vi "CLC_L2_8x8_InPhaseCal_L1_2x2_Auto16AiP.vi"() -> ()   [LabVIEW 2023, in "Clover_Cell.lvlib"]
uses:
  lib/CTL/AiP_index.ctl
  Clover_Cell.lvlib
  lib/Anritsu Signal Analyzer Series/Anritsu Signal Analyzer Series.lvlib
panel:
  out "Numeric":i32
  out "AiP_Change":i32
  out "FileNAME_Dual 2":string
  out "maxPower":dbl
  out "B_Ch_Index":i32[](array[numeric])
  out "A_Ch_Index":i32[](array[numeric])
  out "A-Phase":i32[](array[numeric])
  out "B-Phase":i32[](array[numeric])
  out "Duration(sec)":dbl
  out "Start":u32
  in  "AiP_Base":T1=1 items=["AiP_1"=1, "AiP_2"=2, "AiP_3"=3, "AiP_4"=4, "AiP_5"=5, "AiP_6"=6, "AiP_7"=7, "AiP_8"=8, "AiP_9"=9, "AiP_10"=10, "AiP_11"=11, "AiP_12"=12, "AiP_13"=13, "AiP_14"=14, "AiP_15"=15, "AiP_16"=16]
  in  "WaitingTime":u32=500
  in  "Polarity":u16(ring) items=["H", "V"]
  in  "AvgTimes":i32=5
  in  "TRXmode":u16(ring)=1 items=["Rx"=2, "Tx"=1]
  in  "FileName_Note":string
  out "AiP_Base_Ch":i32
  out "AiP_Change_OFFSetPhase":i32
  out "AiP_Change_Ch":i32
  out "max index\n(OFFSet Step)":i32
  out "trmode":u16
  in  "VISA resource name":refnum<visa-resource-name>="TCPIP0::192.168.100.230::inst0::INSTR"
  out "FileNAME_Dual":string
  out "OK?":bool
  out "output cluster":T2={"address"="192.168.100.111", "remote port or service name"=5025, "timeout ms (60000)"=10000}
  out "SA1":dbl[](graph)
  out "error out":errorcluster
  # "CLC_Gen3_L2_8x8_InPhase_Calibration_by_L1_2x2 Auto"
  # "Setting"
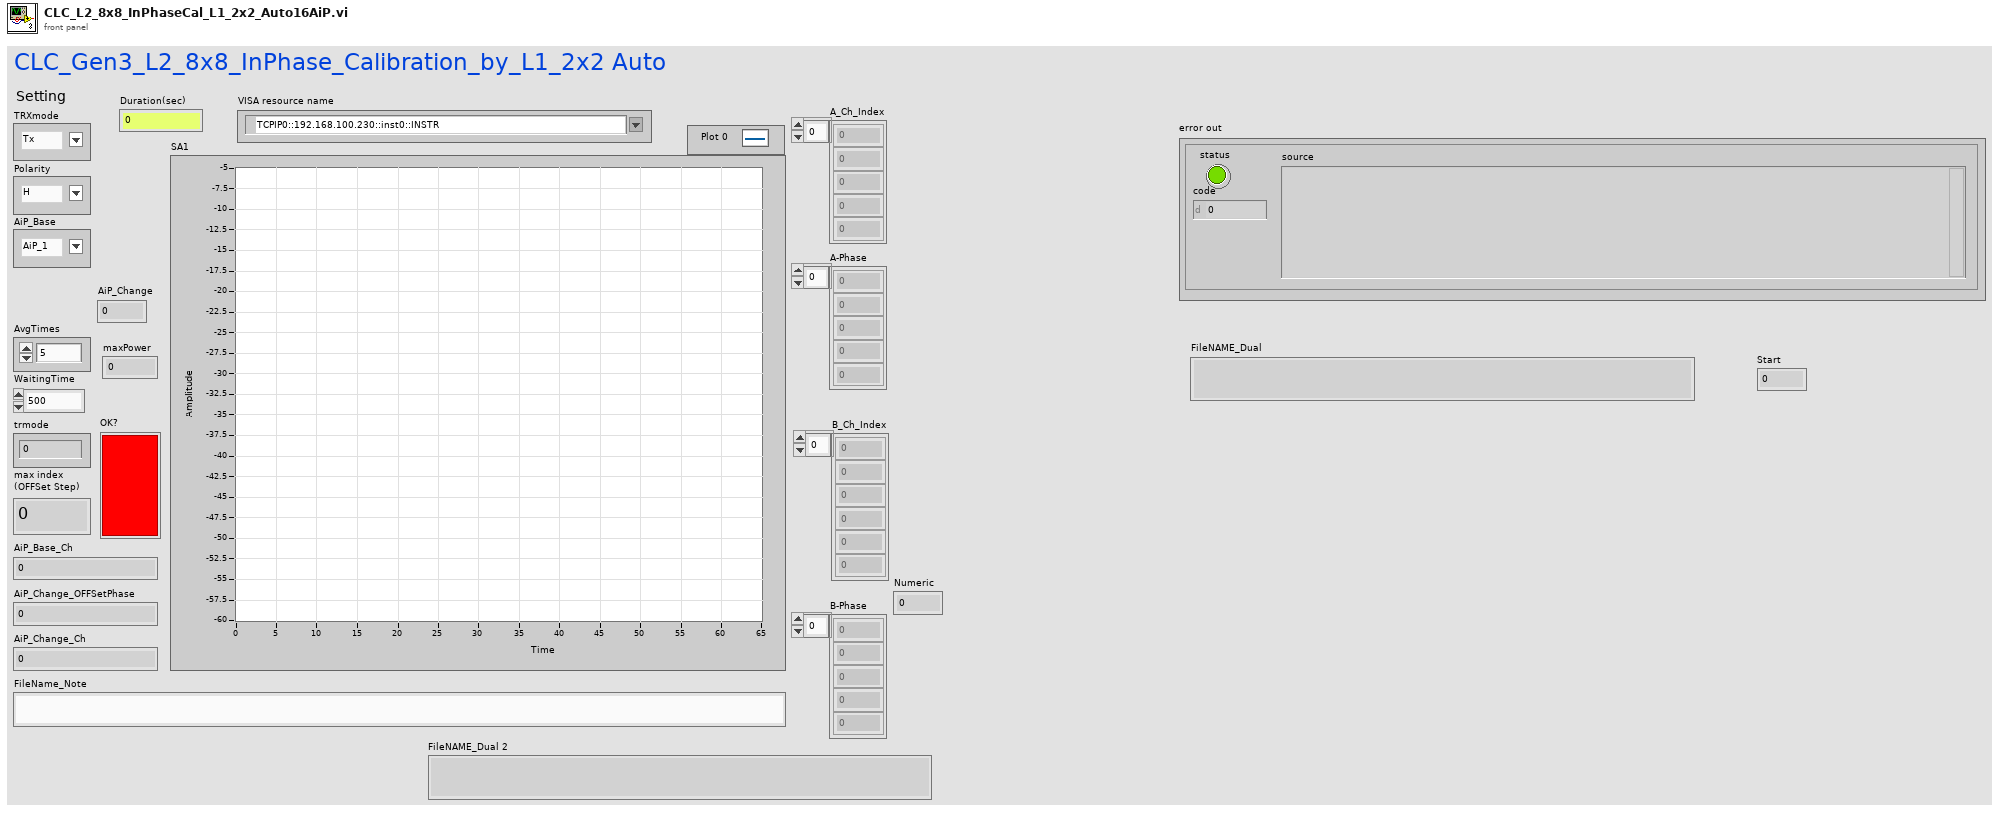
[diagram p1: front panel]
types:
  T1 = typedef "AiP_index.ctl" = u16
  T2 = cluster{"address":string, "remote port or service name":u16, "timeout ms (60000)":i32}
  T3 = cluster{"Mode":u16, "Polarity":u16, "CH_ON/OFF":u16, "Channel":i32, "Gain":i32, "Phase":i32}
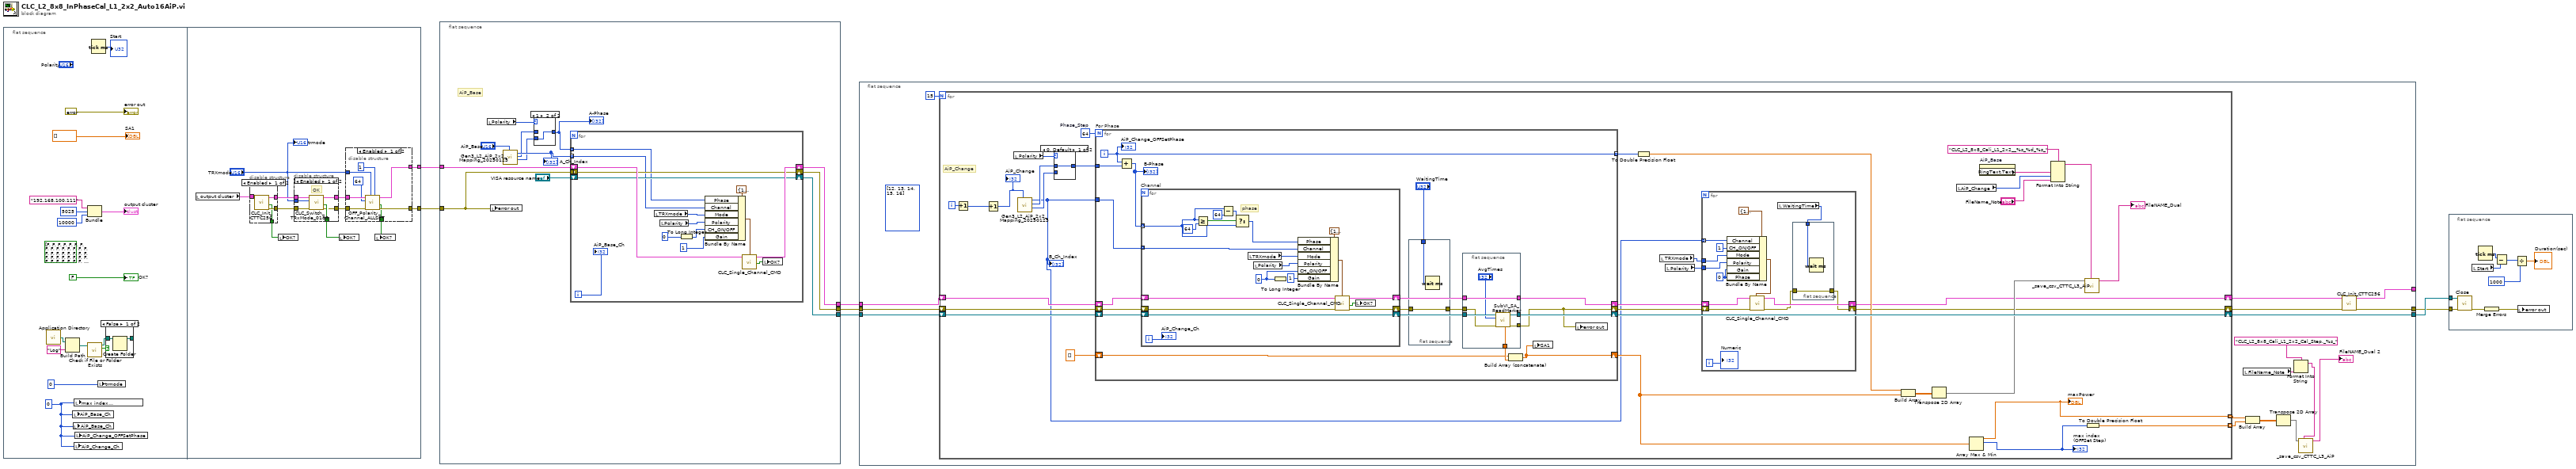
[diagram p0: block diagram]
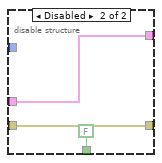
[diagram p5: hidden frame]
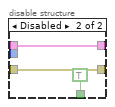
[diagram p6: hidden frame]
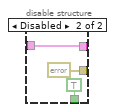
[diagram p7: hidden frame]
diagram:
  n1 = flat-sequence {
    tunnel: [w26] -> w1
    tunnel: [w31] -> w2
    frame #0 {
      w9 = 0 ("max index\n(OFFSet Step)")
      (unwired) bool[][] [[FALSE, FALSE, FALSE, FALSE, FALSE, FALSE, FALSE, FALSE], [FALSE, FALSE, FALSE, FALSE, FALSE, FALSE, FALSE, FALSE], [FALSE, FALSE, FALSE, FALSE, FALSE, FALSE, FALSE, FALSE], [FALSE, FALSE, FALSE, FALSE, FALSE, FALSE, FALSE, FALSE], [FALSE, FALSE, FALSE, FALSE, FALSE, FALSE, FALSE, FALSE], [FALSE, FALSE, FALSE, FALSE, FALSE, FALSE, FALSE, FALSE], [FALSE, FALSE, FALSE, FALSE, FALSE, FALSE, FALSE, FALSE], [FALSE, FALSE, FALSE, FALSE, FALSE, FALSE, FALSE, FALSE]] ("Operating \nChannel(s)")
      n2 = call <vilib>:"Application Directory.vi"() -> ("Application Directory"=w14:path)
      n3 = Build Path(base path=w14, name or relative path="Log") -> (appended path=w11:path)
      n4 = local write "AiP_Base_Ch"(w9) -> ()
      n5 = local write "AiP_Base_Ch"(w9) -> ()
      n6 = local write "AiP_Change_Ch"(w9) -> ()
      n7 = local write "max index\n(OFFSet Step)"(w9) -> ()
      n8 = local write "AiP_Change_OFFSetPhase"(w9) -> ()
      n9 = Bundle("address"="192.168.100.111", "remote port or service name"=u16 5025, "timeout ms (60000)"=10000) -> (→"output cluster":T2)  [unwired: 1 in]
      n10 = call <vilib>:"Check if File or Folder Exists.vi"("path"=w11) -> ("file or folder exists?"=w13:bool, "dup path"=w12:path)  [unwired: 8 in, 1 out]
      n11 = Tick Count (ms)() -> (millisecond timer value=→"Start":u32)
      n12 = local write "trmode"(u16 0 ("trmode")) -> ()
      n13 = case shown="False" w13 {
        tunnel: w12 -> [w24 w25]
        tunnel: [w23 w25] -> _
        frame False {
          n14 = Create Folder(path (use dialog)=w24) -> (created path=w23:path)  [unwired: 2 in, 2 out]
        }
        frame True {
        }
      }
      "error out" <- errorcluster {"status"=FALSE, "code"=0, "source"=""} ("error out")
      "OK?" <- FALSE ("OK?")
      "SA1" <- dbl[] []
    }
    frame #1 {
      n15 = local read "output cluster"() -> (w36:T2)
      n16 = disable-structure shown="Enabled" {
        disable-tunnel: w36 -> [w60 w63]
        disable-tunnel: [w59 w63] -> w35
        disable-tunnel: [w58 errorcluster {"status"=FALSE, "code"=0, "source"=""} ("error in (no error)")] -> w33
        disable-tunnel: [w57 TRUE ("OK?")] -> w28
        frame Enabled {
          n17 = call "CLC_Init_CTTC256.vi"("TCPIPin"=w60) -> ("error out"=w58:errorcluster, "Status"=w57:bool, "TCPIPin 2"=w59:T2)  [unwired: 8 in]
        }
        frame Disabled {
        }
      }
      n18 = local write "OK?"(w28) -> ()
      n19 = disable-structure shown="Enabled" {
        disable-tunnel: w35 -> [w53 w55]
        disable-tunnel: [w52 TRUE ("OK?")] -> w34
        disable-tunnel: w33 -> [w51 w54]
        disable-tunnel: [w50 w54] -> w32
        disable-tunnel: [w49 w55] -> w30
        disable-tunnel: "TRXmode" -> [w48 _]
        frame Enabled {
          # "OK"
          n20 = call "CLC_Switch_TRxMode_0188.vi"("error in (no error)"=w51, "Text Ring"=w48, "TCPIPin"=w53) -> ("error out"=w50:errorcluster, "OK?"=w52:bool, "TCPIPin 2"=w49:T2)  [unwired: 6 in]
        }
        frame Disabled {
        }
      }
      n21 = local write "OK?"(w34) -> ()
      n22 = disable-structure shown="Enabled" {
        disable-tunnel: w32 -> [w44 w46]
        disable-tunnel: [w43 w46] -> w31
        disable-tunnel: w30 -> [w42 w45]
        disable-tunnel: [w41 FALSE ("OK?")] -> w29
        disable-tunnel: "TRXmode" -> [w39 _]
        disable-tunnel: [w37 w45] -> w26
        frame Enabled {
          n23 = call "OFF_Polarity_Channel_ALLSET.vi"("CH_ON:0/OFF:1"=u16 1, "Mode"=w39, "error in"=w44, "Channel"=64, "TCPIPin"=w42) -> ("error out"=w43:errorcluster, "OK?"=w41:bool, "TCPIPout"=w37:T2)  [unwired: 4 in]
        }
        frame Disabled {
        }
      }
      n24 = local write "OK?"(w29) -> ()
      "trmode" <- "TRXmode"
    }
  }
  n25 = flat-sequence {
    tunnel: [w75] -> w7
    tunnel: [w74] -> w6
    tunnel: [w73] -> w5
    tunnel: w2 -> [w72]
    tunnel: w1 -> [w70]
    frame #0 {
      # "AiP_Base"
      n26 = local read "Polarity"() -> (w69:u16)
      n27 = local write "error out"(w72) -> ()
      n28 = call "Gen3_L2_AiP_2x2_Mapping_20250125.vi"("AiP"="AiP_Base") -> ("Pol_V"=w66:i32[], "Pol_H"=w67:i32[], "Ch_Index"=w68:i32[])  [unwired: 8 in]
      "A_Ch_Index" <- w68
      n29 = case shown="1" w69 {
        tunnel: w67 -> [w76 _]
        tunnel: [w76 w77] -> w64
        tunnel: w66 -> [_ w77]
        frame 0, Default {
        }
        frame 1 {
        }
      }
      "A-Phase" <- w64
      n30 = for {
        shift-right: [w89] -> w73
        shift-left: w70 -> [w88]
        tunnel: w72 -> [w83]
        shift-right: [w83] -> w74
        shift-left: _ -> [_]
        shift-right: [w82] -> w75
        shift-left: "VISA resource name" -> [w82]
        tunnel: w68 -> [w81] mode=indexing
        tunnel: w64 -> [w80] mode=indexing
        i -> [w79]
        n31 = local read "TRXmode"() -> (w86:u16)
        n32 = local read "Polarity"() -> (w85:u16)
        n33 = To Long Integer(number=u16 0 ("CH_ON/OFF")) -> (32bit integer=w84:i32)
        n34 = Bundle By Name(cluster=T3 {"Mode"=1, "Polarity"=1, "CH_ON/OFF"=1, "Channel"=0, "Gain"=0, "Phase"=0} ("Channel params"), "Phase"=w80, "Channel"=w81, "Mode"=w86, "Polarity"=w85, "CH_ON/OFF"=w84, "Gain"=1) -> (w92:T3)
        n35 = call "CLC_Single_Channel_CMD.vi"("Channel params"=w92, "TCPIPin"=w88) -> ("OK?"=w91:bool, "TCPIPout"=w89:T2)  [unwired: 7 in, 1 out]
        n36 = local write "OK?"(w91) -> ()
        "AiP_Base_Ch" <- w79
      }
    }
  }
  n37 = flat-sequence {
    tunnel: w7 -> [w109]
    tunnel: w6 -> [w108]
    tunnel: w5 -> [w107]
    tunnel: [w106] -> w4
    tunnel: [w104] -> w3
    tunnel: [w105] -> _
    frame #0 {
      (unwired) i32[] [12, 13, 14, 15, 16]
      n38 = for {
        N: 15 -> [_]
        shift-right: [w139] -> w106
        shift-left: w109 -> [w143]
        shift-right: [w120] -> w102
        shift-left: w108 -> [w142]
        shift-right: [w121] -> w103
        shift-left: w107 -> [w141]
        tunnel: [w119] -> w96 mode=indexing
        tunnel: [w117] -> w95 mode=indexing
        i -> [w115]
        w138 = 64  # Phase_Step
        # "AiP_Change"
        n39 = Increment(x=w115) -> (x+1=w116:i32)
        n40 = Increment(x=w116) -> (x+1=w110:i32)
        "AiP_Change" <- w110
        n41 = local read "Polarity"() -> (w136:u16)
        n42 = call "Gen3_L2_AiP_2x2_Mapping_20250125.vi"("AiP"=w110) -> ("Pol_V"=w134:i32[], "Pol_H"=w135:i32[], "Ch_Index"=w111:i32[])  [unwired: 8 in]
        "B_Ch_Index" <- w111
        n43 = case shown="0, Default" w136 {
          tunnel: w135 -> [w160 _]
          tunnel: [w160 w161] -> w133
          tunnel: w134 -> [_ w161]
          frame 0, Default {
          }
          frame 1 {
          }
        }
        n44 = for "For Phase" {
          N: w138 -> [_]
          shift-right: [w173] -> w122
          shift-left: w141 -> [w175]
          shift-right: [w172] -> w123
          shift-left: w142 -> [w176]
          shift-right: [w179] -> w139
          shift-left: w143 -> [w170]
          shift-right: [w174] -> w132
          shift-left: dbl[] [] -> [w177]
          tunnel: w111 -> [w168]
          tunnel: w133 -> [w167]
          tunnel: [w165] -> w131 mode=indexing
          i -> [w165]
          n45 = Add(x=w165, y=w167) -> (x+y=w166:i32[])
          "B-Phase" <- w166
          n46 = for "Channel" {
            shift-right: [w191] -> w164
            shift-left: w176 -> [w196]
            shift-right: [w192] -> w171
            shift-left: w175 -> [w195]
            shift-right: [w190] -> w169
            shift-left: w170 -> [w190]
            tunnel: w168 -> [w189] mode=indexing
            tunnel: w166 -> [w184] mode=indexing
            i -> [w182]
            w200 = u16 0 ("CH_ON/OFF")
            # "phase"
            n47 = Greater Or Equal?(x=w184, y=64) -> (x >= y?=w187:bool)
            n48 = Subtract(x=w184, y=64) -> (x-y=w188:i32)
            n49 = Select(t=w188, s=w187, f=w184) -> (s? t:f=w183:i32)
            n50 = local read "TRXmode"() -> (w198:u16)
            n51 = local read "Polarity"() -> (w199:u16)
            n52 = To Long Integer(number=w200) -> ()  [unwired: 1 out]
            n53 = Bundle By Name(cluster=T3 {"Mode"=1, "Polarity"=1, "CH_ON/OFF"=1, "Channel"=0, "Gain"=0, "Phase"=0} ("Channel params"), "Phase"=w183, "Channel"=w189, "Mode"=w198, "Polarity"=w199, "CH_ON/OFF"=w200, "Gain"=1) -> (w193:T3)
            n54 = call "CLC_Single_Channel_CMD.vi"("Channel params"=w193, "error in"=w196, "TCPIPin"=w195) -> ("error out"=w191:errorcluster, "OK?"=w194:bool, "TCPIPout"=w192:T2)  [unwired: 6 in]
            n55 = local write "OK?"(w194) -> ()
            "AiP_Change_Ch" <- w182
          }
          n56 = flat-sequence {
            tunnel: w164 -> [w181]
            tunnel: [w181] -> w163
            tunnel: "WaitingTime" -> [w180]
            frame #0 {
              n57 = Wait (ms)(milliseconds to wait=w180) -> ()  [unwired: 1 out]
            }
          }
          n58 = flat-sequence {
            tunnel: [w208] -> w179
            tunnel: [w207] -> w178
            tunnel: [w206] -> w172
            tunnel: w169 -> [w205]
            tunnel: w163 -> [w204]
            tunnel: [w203] -> w173
            tunnel: w171 -> [w203]
            frame #0 {
              n59 = call "SubVI_SA_ReadMarker.vi"("error in (no error)"=w204, "AvgTimes"="AvgTimes", "VISA resource name"=w205) -> ("error out"=w206:errorcluster, "VISA resource name out"=w208:refnum<visa-resource-name>, "Marker Power"=w207:dbl)  [unwired: 5 in, 1 out]
            }
          }
          n60 = Build Array (concatenate)(w177, w178) -> (w174:dbl[])
          n61 = local write "SA1"(w174) -> ()
          n62 = local write "error out"(w172) -> ()
          "AiP_Change_OFFSetPhase" <- w165
        }
        n63 = To Double Precision Float(number=w131) -> (double precision float=w130:dbl[])
        n64 = local read "TRXmode"() -> (w113:u16)
        n65 = local read "Polarity"() -> (w112:u16)
        n66 = for {
          shift-right: [w155] -> w121
          shift-left: w122 -> [w156]
          shift-right: [w146] -> w120
          shift-left: w123 -> [w157]
          tunnel: w111 -> [w154] mode=indexing
          tunnel: w113 -> [w149]
          tunnel: w112 -> [w148]
          i -> [w153]
          w150 = 0 ("Phase")
          n67 = Bundle By Name(cluster=T3 {"Mode"=1, "Polarity"=1, "CH_ON/OFF"=0, "Channel"=11, "Gain"=1, "Phase"=43} ("Channel params"), "Channel"=w154, "CH_ON/OFF"=u16 1, "Mode"=w149, "Polarity"=w148, "Gain"=w150, "Phase"=w150) -> (w151:T3)
          n68 = call "CLC_Single_Channel_CMD.vi"("Channel params"=w151, "error in"=w157, "TCPIPin"=w156) -> ("error out"=w147:errorcluster, "TCPIPout"=w155:T2)  [unwired: 6 in, 1 out]
          n69 = local read "WaitingTime"() -> (w145:u32)
          n70 = flat-sequence {
            tunnel: w147 -> [w159]
            tunnel: [w159] -> w146
            tunnel: w145 -> [w158]
            frame #0 {
              n71 = Wait (ms)(milliseconds to wait=w158) -> ()  [unwired: 1 out]
            }
          }
          "Numeric" <- w153
        }
        n72 = Build Array(w130, w132) -> (w140:dbl[][])
        n73 = Transpose 2D Array(2D array=w140) -> (transposed array=w124:dbl[][])
        n74 = local read "AiP_Change"() -> (w114:i32)
        n75 = Array Max & Min(array=w132) -> (max value=w119:dbl, max index (indices)=w118:i32)  [unwired: 2 out]
        "max index\n(OFFSet Step)" <- w118
        "maxPower" <- w119
        n76 = property on="AiP_Base" class="Ring (strict)"() -> ("RingText.Text"=w128:string)  [unwired: 2 in, 2 out]
        n77 = Format Into String(format string="CLC_L2_8x8_Cali_L1_2x2__%s_%d_%s_", w128, w114, "FileName_Note") -> (resulting string=w127:string)  [unwired: 2 in, 1 out]
        n78 = call "_save_csv_CTTC_L3_AiP.vi"("delimiter (\\t)"=w127, "Data"=w124) -> ("FileName"=→"FileNAME_Dual":string)  [unwired: 9 in]
        n79 = To Double Precision Float(number=w118) -> (double precision float=w117:dbl)
      }
      n80 = local read "FileName_Note"() -> (w99:string)
      n81 = Build Array(w96, w95) -> (w97:dbl[][])
      n82 = Transpose 2D Array(2D array=w97) -> (transposed array=w94:dbl[][])
      n83 = Format Into String(format string="CLC_L2_8x8_Cali_L1_2x2_Cal_Step._%s_", w99) -> (resulting string=w98:string)  [unwired: 2 in, 1 out]
      n84 = call "_save_csv_CTTC_L3_AiP.vi"("delimiter (\\t)"=w98, "Data"=w94) -> ("FileName"=→"FileNAME_Dual 2":string)  [unwired: 9 in]
      n85 = call "CLC_Init_CTTC256.vi"("error in (no error)"=w102, "TCPIPin"=w103) -> ("error out"=w104:errorcluster, "TCPIPin 2"=w105:T2)  [unwired: 7 in, 1 out]
    }
  }
  n86 = flat-sequence {
    tunnel: w4 -> [w216]
    tunnel: w3 -> [w215]
    frame #0 {
      n87 = call "Close.vi"("error in (no error)"=w215, "VISA resource name"=w216) -> ("error out"=w217:errorcluster)  [unwired: 9 in]
      n88 = local read "Start"() -> (w212:u32)
      n89 = Tick Count (ms)() -> (millisecond timer value=w213:u32)
      n90 = Merge Errors(w217) -> (w214:errorcluster)
      n91 = Subtract(x=w213, y=w212) -> (x-y=w211:u32)
      n92 = Divide(x=w211, y=u32 1000) -> (x/y=→"Duration(sec)":dbl)
      n93 = local write "error out"(w214) -> ()
    }
  }
